vi "Register Settings Update.vi"(8 "error in (no error)":errorcluster, 11 "Instr in":refnum<class "Instrument.lvclass">) -> (0 "error out":errorcluster, 3 "Instr out":refnum<class "Instrument.lvclass">)   [LabVIEW 2014, in "Instrument.lvclass"]
uses:
  Instrument.lvclass
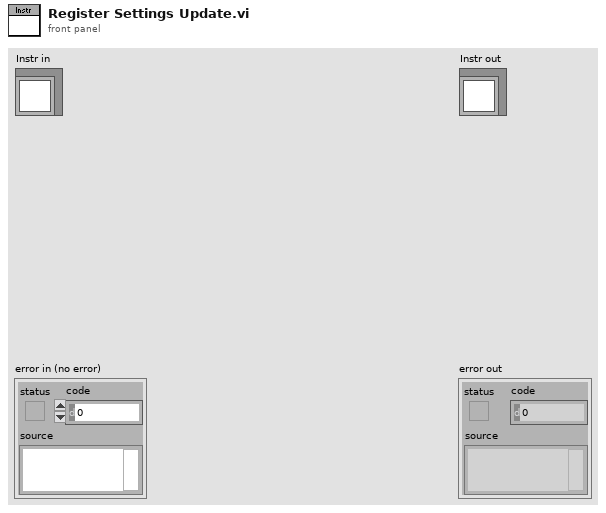
[diagram p1: front panel]
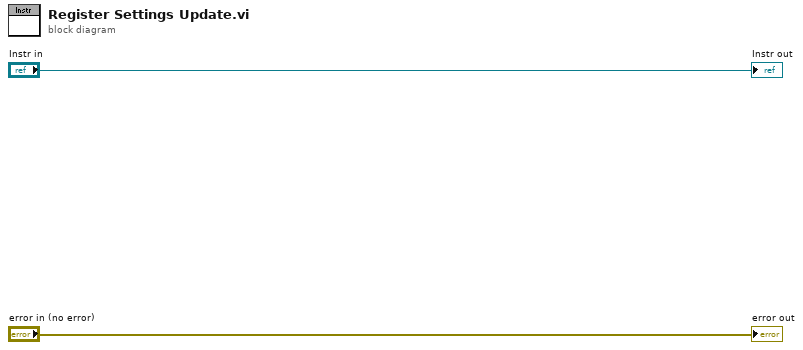
[diagram p0: block diagram]
diagram:
  "error out" <- "error in (no error)"
  "Instr out" <- "Instr in"
